vi "Ph_prep_to_plot.vi"(1 "Ph":i32[][](array[numeric])) -> (0 "Array":cluster{"Ph":i32[], dbl[]}[](array[cluster]))   [LabVIEW 2010]
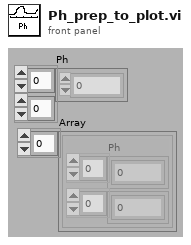
[diagram p1: front panel]
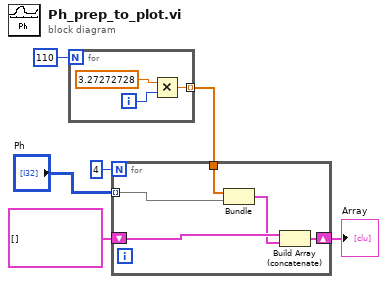
[diagram p0: block diagram]
diagram:
  n1 = for {
    N: 110 -> [_]
    tunnel: [w7] -> w1 mode=indexing
    i -> [w8]
    n2 = Multiply(x=3.27272728, y=w8) -> (x*y=w7:dbl)
  }
  n3 = for {
    N: 4 -> [_]
    tunnel: "Ph" -> [w11] mode=indexing
    shift-right: [w13] -> w4
    shift-left: cluster{dbl[], "Ph":i32[]}[] [] -> [w14]
    tunnel: w1 -> [w10]
    n4 = Bundle(w10, "Ph"=w11) -> (w12:cluster{dbl[], "Ph":i32[]})  [unwired: 1 in]
    n5 = Build Array (concatenate)(w14, w12) -> (w13:cluster{dbl[], "Ph":i32[]}[])
  }
  "Array" <- w4
